vi "checkworking.vi"(1 "Array":bool[](array[boolean])) -> (9 "Boolean":bool)   [LabVIEW 2012]
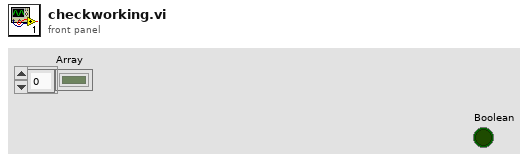
[diagram p1: front panel]
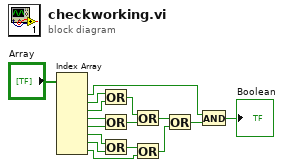
[diagram p0: block diagram]
diagram:
  n1 = Index Array(array="Array") -> (element #1=w1:bool, element #2=w8:bool, element #3=w7:bool, element #4=w6:bool, element #5=w5:bool, element #6=w4:bool, element #7=w3:bool, element #8=w2:bool)  [unwired: 8 in]
  n2 = Or(x=w8, y=w7) -> (x .or. y?=w16:bool)
  n3 = Or(x=w6, y=w5) -> (x .or. y?=w15:bool)
  n4 = Or(x=w4, y=w3) -> (x .or. y?=w14:bool)
  n5 = Or(x=w16, y=w15) -> (x .or. y?=w13:bool)
  n6 = Or(x=w14, y=w2) -> (x .or. y?=w12:bool)
  n7 = Or(x=w13, y=w12) -> (x .or. y?=w11:bool)
  n8 = And(x=w1, y=w11) -> (x .and. y?=→"Boolean":bool)
